vi "P_Stat_Status1.vi"(8 "error in (no error)":errorcluster, 11 ".NET Refnum in":refnum<k24>) -> (0 "error out":errorcluster, 1 "PotentialOverload":bool, 2 "ManualCellSwitch":bool, 3 "Oscillation":bool, 4 "TemperatureOverload":bool, 5 "CurrentOverload":bool, 7 "Cell":bool)   [LabVIEW 2020]
uses:
  C:/Users/Benj/Desktop/SEC Software V4.9/EcoChemie.Autolab.Sdk.dll
  SEC Software V4.9/EcoChemie.Autolab.Sdk.dll
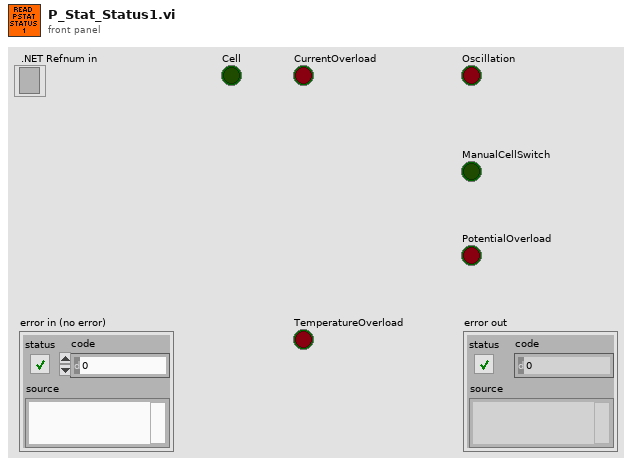
[diagram p1: front panel]
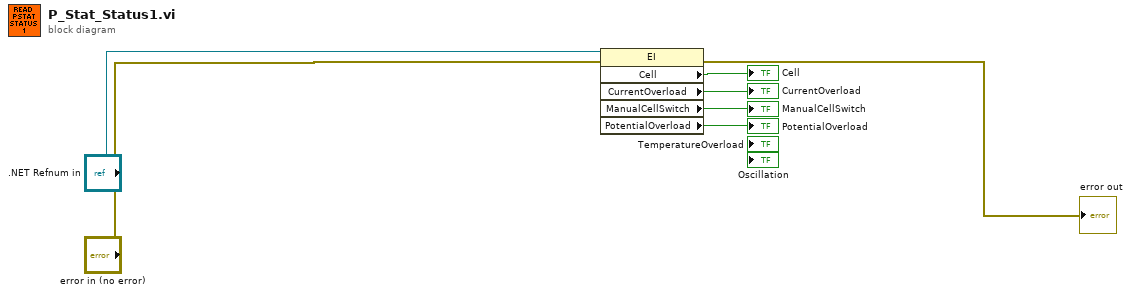
[diagram p0: block diagram]
diagram:
  n1 = property class="EI"(reference=".NET Refnum in", error in="error in (no error)") -> (error out=→"error out":errorcluster, "Cell"=→"Cell":bool, "CurrentOverload"=→"CurrentOverload":bool, "ManualCellSwitch"=→"ManualCellSwitch":bool, "PotentialOverload"=→"PotentialOverload":bool)  [unwired: 1 out]
